vi "Get_Fast_FID_Calibrations.vi"(1 "Code Name":string, 2 "Calib File String":string, 3 "Take New Data":bool) -> (0 "Calib Constants":dbl[](array[numeric]) format="%.6f")   [LabVIEW 2010]
uses:
  Globals/Meas_global.vi
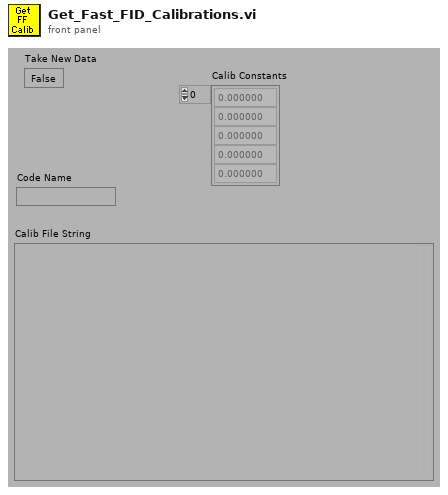
[diagram p1: front panel]
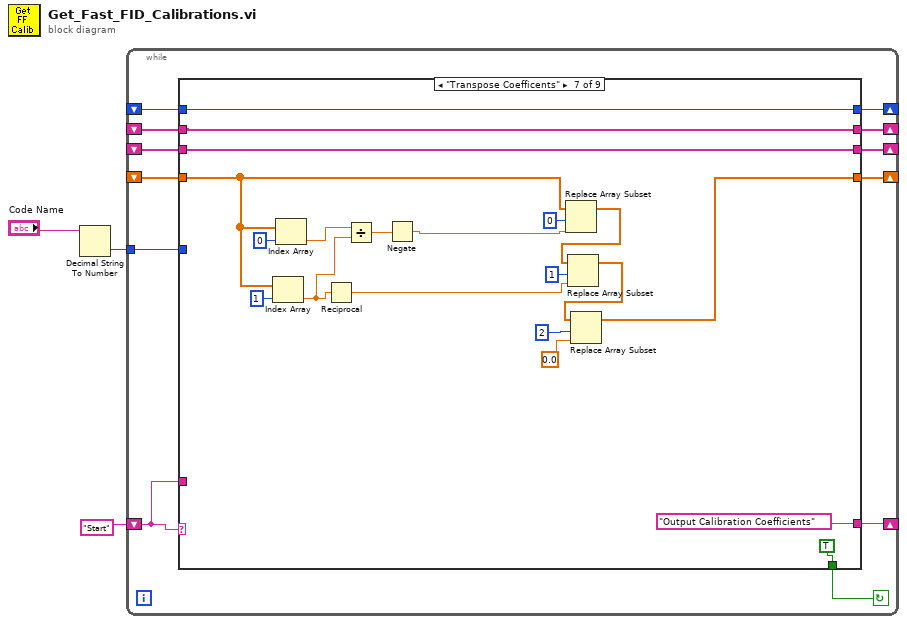
[diagram p0: block diagram]
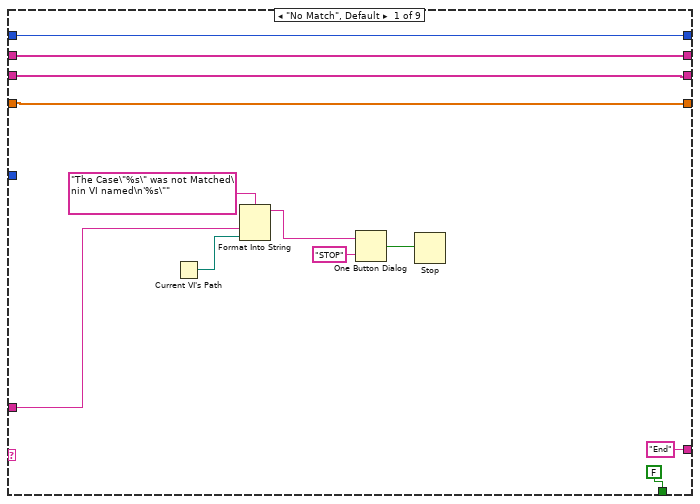
[diagram p2: hidden frame]
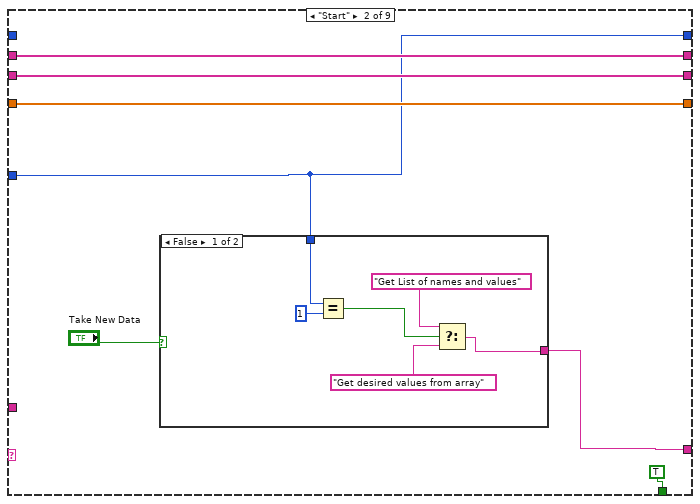
[diagram p3: hidden frame]
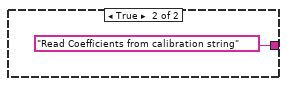
[diagram p4: hidden frame]
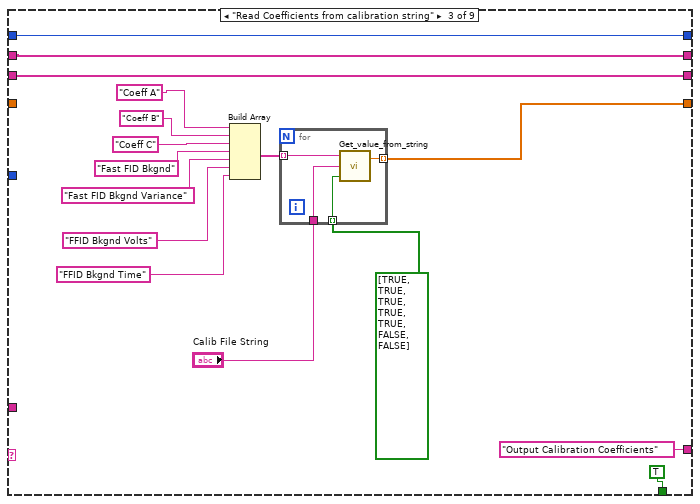
[diagram p5: hidden frame]
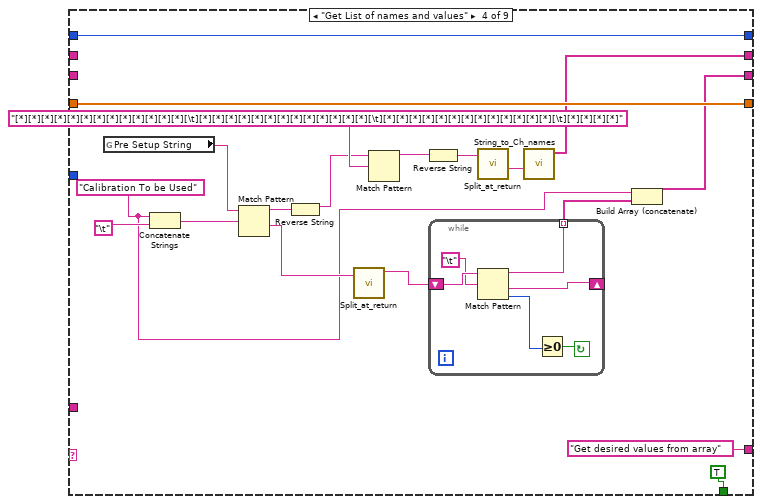
[diagram p6: hidden frame]
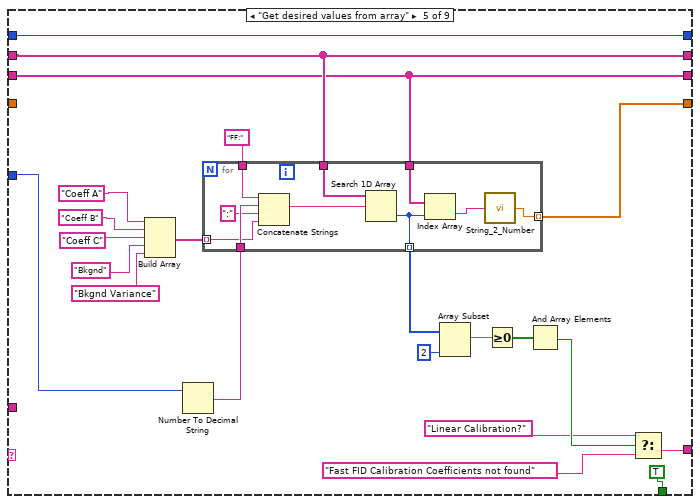
[diagram p7: hidden frame]
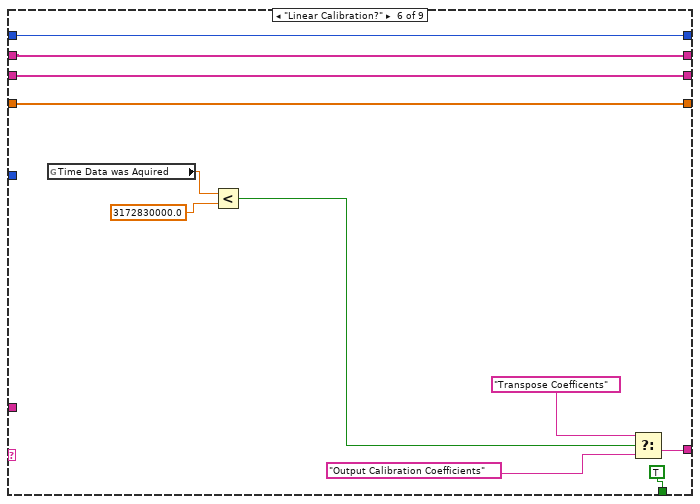
[diagram p8: hidden frame]
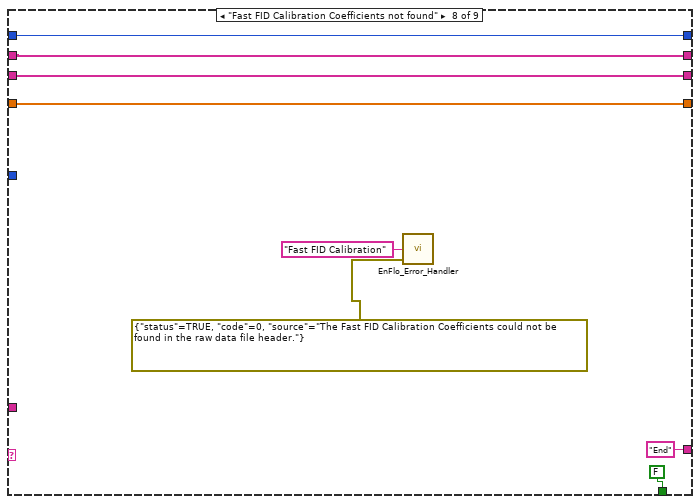
[diagram p9: hidden frame]
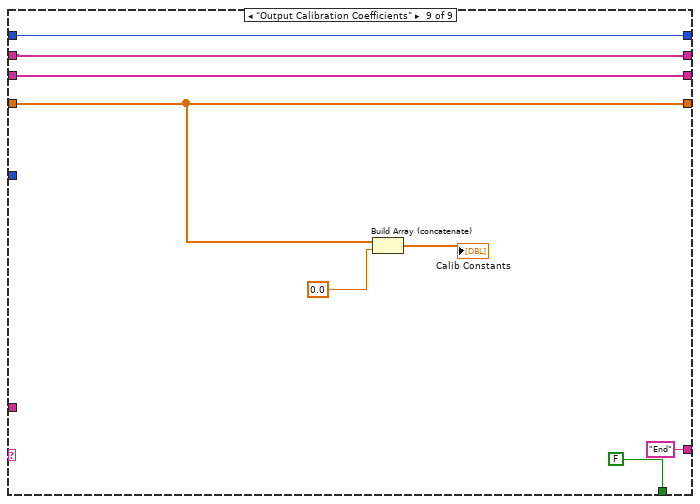
[diagram p10: hidden frame]
diagram:
  n1 = Decimal String To Number(string="Code Name") -> (number=w1:i32)  [unwired: 3 out]
  n2 = while {
    shift-left: _ -> [w10]
    shift-right: [w9] -> _
    shift-left: _ -> [w11]
    shift-right: [w12] -> _
    shift-left: _ -> [w14]
    shift-right: [w13] -> _
    shift-left: "Start" -> [w7]
    shift-right: [w15] -> _
    shift-right: [w6] -> _
    shift-left: _ -> [w5]
    tunnel: w1 -> [w4]
    stop <- w8 continue-if-true
    n3 = case shown="\"Transpose Coefficents\"" w7 {
      tunnel: ["End" w31 "Output Calibration Coefficients" "Get desired values from array" w90 w123 "Output Calibration Coefficients" "End" "End"] -> w15
      tunnel: w14 -> [w17 w34 _ w78 _ w119 w139 w150 w164]
      tunnel: [w17 w34 w56 w78 w98 w119 w136 w150 w164] -> w13
      tunnel: w11 -> [w18 w33 w55 _ w99 w126 w146 w154 w163]
      tunnel: [w18 w33 w55 w63 w99 w126 w146 w154 w163] -> w12
      tunnel: w10 -> [w19 _ w54 w80 w107 w128 w148 w156 w162]
      tunnel: [w19 w28 w54 w80 w107 w128 w148 w156 w162] -> w9
      tunnel: [FALSE TRUE TRUE TRUE TRUE TRUE TRUE FALSE FALSE] -> w8
      tunnel: w7 -> [w22 _ _ _ _ _ _ _ _]
      tunnel: [w16 w29 w53 w67 w100 w127 w147 w155 w160] -> w6
      tunnel: w5 -> [w16 w29 w53 _ w100 w127 w147 w155 w160]
      tunnel: w4 -> [_ w28 _ _ w101 _ _ _ _]
      frame "No Match", Default {
        n4 = Current VI's Path() -> (path=w23:path)
        n5 = Format Into String(format string="The Case\"%s\" was not Matched\nin VI named\n'%s\"" ("Format String"), w22, w23) -> (resulting string=w26:string)  [unwired: 2 in, 1 out]
        n6 = One Button Dialog(message=w26, button name ("OK")="STOP") -> (true=w24:bool)
        n7 = Stop(stop? (T)=w24) -> ()
      }
      frame "Start" {
        n8 = case shown="False" "Take New Data" {
          tunnel: [w37 "Read Coefficients from calibration string"] -> w31
          tunnel: w28 -> [w40 _]
          frame False {
            n9 = Equal?(x=w40, y=1) -> (x = y?=w38:bool)
            n10 = Select(t="Get List of names and values", s=w38, f="Get desired values from array") -> (s? t:f=w37:string)
          }
          frame True {
          }
        }
      }
      frame "Read Coefficients from calibration string" {
        n11 = Build Array("Coeff A", "Coeff B", "Coeff C", "Fast FID Bkgnd", "Fast FID Bkgnd Variance", "FFID Bkgnd Volts", "FFID Bkgnd Time") -> (w48:string[])
        n12 = for {
          tunnel: w48 -> [w61] mode=indexing
          tunnel: "Calib File String" -> [w60]
          tunnel: [w59] -> w56 mode=indexing
          tunnel: bool[] [TRUE, TRUE, TRUE, TRUE, TRUE, FALSE, FALSE] ("appended array") -> [w58] mode=indexing
          n13 = call "Get_value_from_string.vi"("Show Dialog?"=w58, "Input string"=w60, "Variable name"=w61) -> ("Value"=w59:dbl)  [unwired: 1 out]
        }
      }
      frame "Get List of names and values" {
        w62 = "Calibration To be Used" ("Input Element")
        n14 = global read "Meas_global.vi" "Pre Setup String"() -> (w75:string)
        n15 = Concatenate Strings(w62, "\t") -> (w76:string)
        n16 = Match Pattern(string=w75, regular expression=w76) -> (before substring=w74:string, after substring=w68:string)  [unwired: 3 out]
        n17 = Reverse String(1:w74) -> (0:w72:string)
        n18 = call "Split_at_return.vi"("String"=w68) -> ("before substring"=w79:string)  [unwired: 1 in, 3 out]
        n19 = Match Pattern(string=w72, regular expression="[*][*][*][*][*][*][*][*][*][*][*][*][*][\t][*][*][*][*][*][*][*][*][*][*][*][*][*][\t][*][*][*][*][*][*][*][*][*][*][*][*][*][\t][*][*][*][*]" ("String")) -> (before substring=w71:string)  [unwired: 4 out]
        n20 = Reverse String(1:w71) -> (0:w70:string)
        n21 = while {
          tunnel: [w81] -> w64 mode=indexing
          shift-left: w79 -> [w86]
          shift-right: [w82] -> _
          stop <- w83 continue-if-true
          n22 = Match Pattern(string=w86, regular expression="\t") -> (before substring=w81:string, after substring=w82:string, offset past match=w84:i32)  [unwired: 2 out]
          n23 = Greater Or Equal To 0?(x=w84) -> (x >= 0?=w83:bool)
        }
        n24 = call "Split_at_return.vi"("String"=w70) -> ("after substring"=w69:string)  [unwired: 1 in, 3 out]
        n25 = call "String_to_Ch_names.vi"("Spreadsheet string"=w69) -> ("Ch names"=w67:string[])  [unwired: 3 out]
        n26 = Build Array (concatenate)(w62, w64) -> (w63:string[])
      }
      frame "Get desired values from array" {
        n27 = Build Array("Coeff A", "Coeff B", "Coeff C", "Bkgnd", "Bkgnd Variance") -> (w103:string[])
        n28 = Number To Decimal String(number=w101) -> (decimal integer string=w104:string)  [unwired: 1 out]
        n29 = for {
          tunnel: "FF:" -> [w118]
          tunnel: w104 -> [w117]
          tunnel: w103 -> [w115] mode=indexing
          tunnel: w100 -> [w114]
          tunnel: w99 -> [w112]
          tunnel: [w110] -> w98 mode=indexing
          tunnel: [w109] -> w97 mode=indexing
          n30 = Concatenate Strings(w118, w117, ":" ("Substring"), w115) -> (w113:string)
          n31 = Search 1D Array(1D array=w114, element=w113) -> (index of element=w109:i32)  [unwired: 1 out]
          n32 = Index Array(array=w112, index=w109) -> (element=w111:string)
          n33 = call "String_2_Number.vi"("Value"=w111) -> ("Numeric"=w110:dbl)
        }
        n34 = Array Subset(array=w97, length=2) -> (w95:i32[])  [unwired: 1 in]
        n35 = Greater Or Equal To 0?(x=w95) -> (x >= 0?=w94:bool[])
        n36 = And Array Elements(Boolean array=w94) -> (logical AND=w93:bool)
        n37 = Select(t="Linear Calibration?", s=w93, f="Fast FID Calibration Coefficients not found") -> (s? t:f=w90:string)
      }
      frame "Linear Calibration?" {
        n38 = global read "Meas_global.vi" "Time Data was Aquired"() -> (w122:dbl)
        n39 = Less?(x=w122, y=3172830000.0 ("double precision float")) -> (x < y?=w120:bool)
        n40 = Select(t="Transpose Coefficents", s=w120, f="Output Calibration Coefficients") -> (s? t:f=w123:string)
      }
      frame "Transpose Coefficents" {
        n41 = Index Array(array=w139, index=1) -> (element=w132:dbl)
        n42 = Index Array(array=w139, index=0) -> (element=w133:dbl)
        n43 = Reciprocal(x=w132) -> (1/x=w134:dbl)
        n44 = Divide(x=w133, y=w132) -> (x/y=w131:dbl)
        n45 = Negate(x=w131) -> (-x=w130:dbl)
        n46 = Replace Array Subset(array=w139, new element=w130, index=0) -> (w138:dbl[])
        n47 = Replace Array Subset(array=w138, new element=w134, index=1) -> (w137:dbl[])
        n48 = Replace Array Subset(array=w137, new element=0.0 ("new element/subarray"), index=2) -> (w136:dbl[])
      }
      frame "Fast FID Calibration Coefficients not found" {
        n49 = call "EnFlo_Error_Handler.vi"("error in (no error)"=errorcluster {"status"=TRUE, "code"=0, "source"="The Fast FID Calibration Coefficients could not be found in the raw data file header."}, "Error Type"="Fast FID Calibration") -> ()  [unwired: 1 in, 3 out]
      }
      frame "Output Calibration Coefficients" {
        n50 = Build Array (concatenate)(w164, 0.0) -> (→"Calib Constants":dbl[])
      }
    }
  }
